vi "GenerateRandomWord.vi"(0 "Controller in":refnum<class "Controller.lvclass">, 3 "error in (no error)":errorcluster) -> (7 "Controller out":refnum<class "Controller.lvclass">, 8 "Word":string, 10 "error out":errorcluster)   [LabVIEW 2024, in "GUI.lvlib" / "Controller.lvclass"]
uses:
  Controller.lvclass
  Controller.lvclass/Controller.ctl
  <vilib>/httpClient/LabVIEWHTTPClient.lvlib
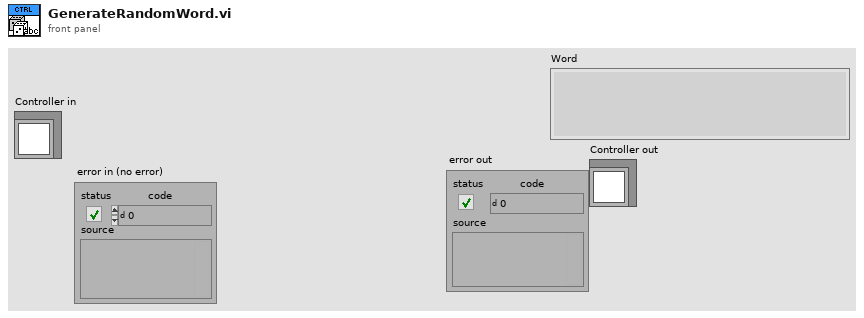
[diagram p1: front panel]
types:
  T1 = typedef "LabVIEWHTTPClient.lvlib/ClientHandle.ctl" = refnum<k1>
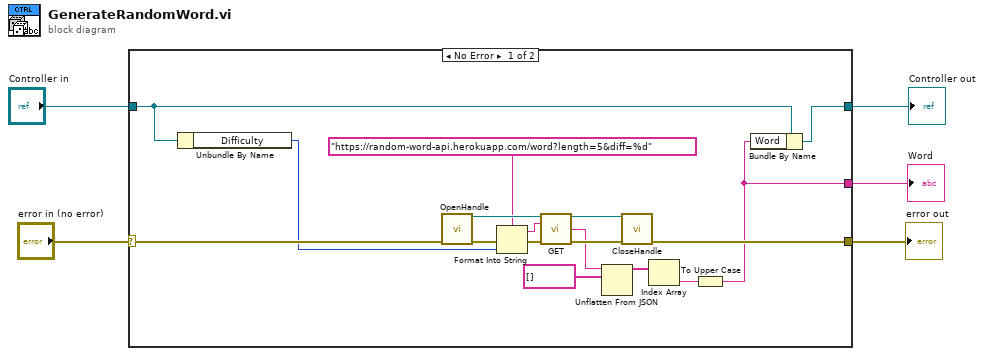
[diagram p0: block diagram]
diagram:
  n1 = case shown="No Error" "error in (no error)" {
    selector: "error in (no error)" -> [w15 w24]
    tunnel: [w10 _] -> w5
    tunnel: [w19 w24] -> w4
    tunnel: "Controller in" -> [w12 w23]
    tunnel: [w13 w23] -> w1
    frame No Error {
      n2 = Unbundle By Name(w12) -> ("Difficulty"=w11:i32)
      n3 = call <vilib>:"OpenHandle.vi"("error in (no error)"=w15) -> ("client handle out"=w22:T1, "error out"=w17:errorcluster)  [unwired: 13 in]
      n4 = Format Into String(format string="https://random-word-api.herokuapp.com/word?length=5&diff=%d" ("url"), error in=w17, w11) -> (resulting string=w14:string, error out=w16:errorcluster)  [unwired: 1 in]
      n5 = call <vilib>:"GET.vi"("client handle"=w22, "url"=w14, "error in (no error)"=w16) -> ("client handle out"=w21:T1, "body"=w9:string, "error out"=w20:errorcluster)  [unwired: 9 in, 1 out]
      n6 = Unflatten From JSON(JSON string=w9, type and defaults=string[] []) -> (value=w7:string[])  [unwired: 5 in, 1 out]
      n7 = call <vilib>:"CloseHandle.vi"("client handle"=w21, "error in (no error)"=w20) -> ("error out"=w19:errorcluster)  [unwired: 13 in]
      n8 = Index Array(array=w7) -> (element=w6:string)  [unwired: 1 in]
      n9 = To Upper Case(1:w6) -> (0:w10:string)
      n10 = Bundle By Name(cluster=w12, "Word"=w10) -> (w13:refnum<class "Controller.lvclass">)
    }
    frame Error {
    }
  }
  "Word" <- w5
  "error out" <- w4
  "Controller out" <- w1
